vi "ultima aula labview.vi"() -> ()   [LabVIEW 2024]
uses:
  <vilib>/Instr/_visa.llb/VISA Configure Serial Port (Instr).vi
panel:
  out "output 2":dbl
  out "output 1":dbl
  out "Temperature":dbl(graph)
  out "Humicity":dbl(graph)
  in  "termination char\n(0xA = '\\n' = LF)":u8=10 format="%.0x"
  out "read buffer":string
  in  "Numeric":dbl
  in  "VISA resource name":refnum<visa-resource-name>
  in  "String":string
  in  "stop":bool
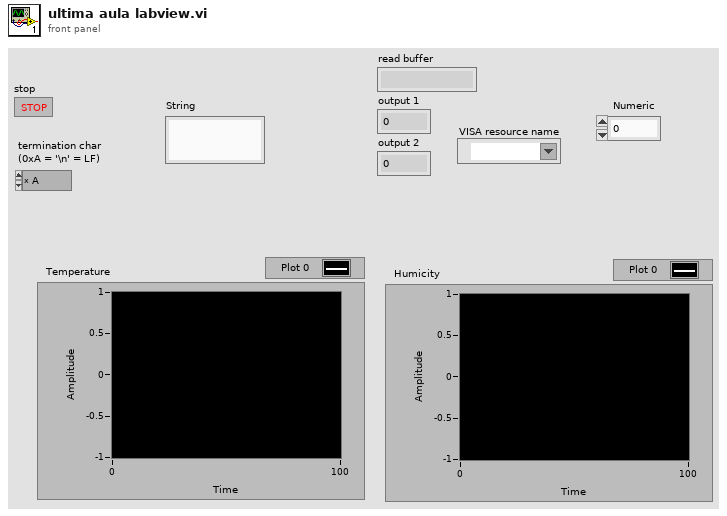
[diagram p1: front panel]
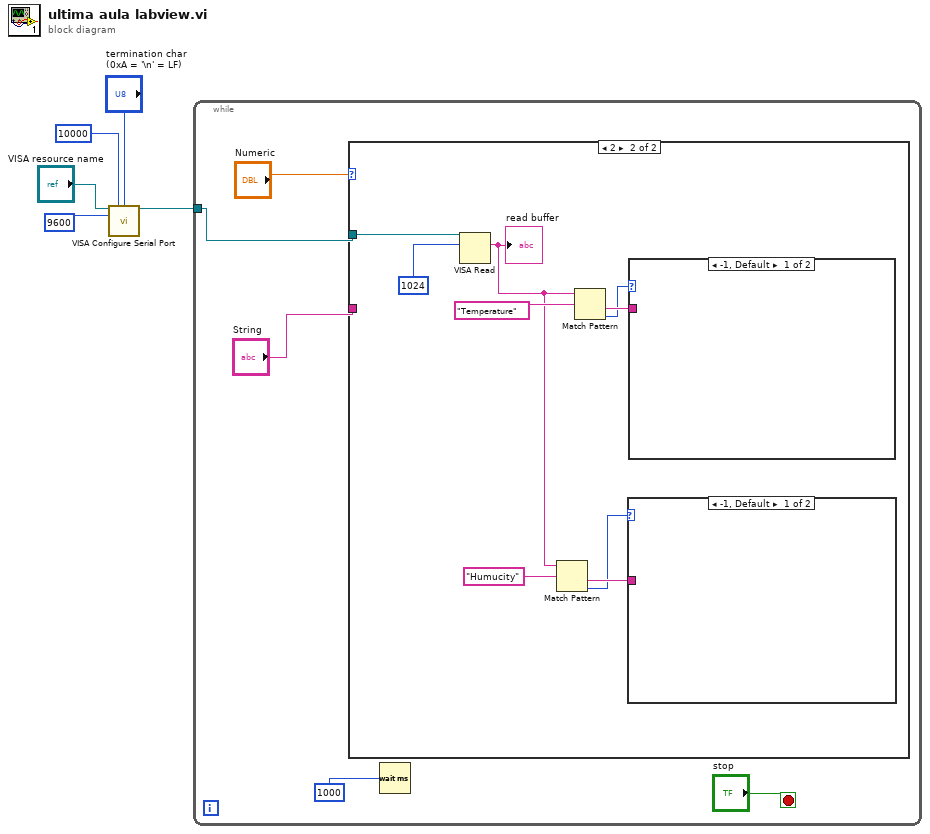
[diagram p0: block diagram]
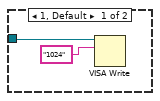
[diagram p2: hidden frame]
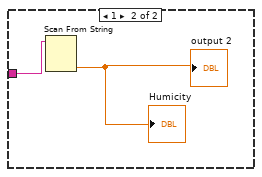
[diagram p3: hidden frame]
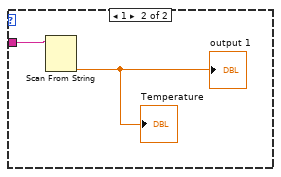
[diagram p4: hidden frame]
diagram:
  n1 = call-poly "VISA Configure Serial Port"("VISA resource name"="VISA resource name", "timeout (10sec)"=u32 10000, "termination char\n(0xA = '\\n' = LF)"="termination char\n(0xA = '\\n' = LF)", "baud rate (9600)"=u32 9600) -> ("VISA resource name out"=w4:refnum<visa-resource-name>)  [unwired: 10 in, 1 out]
  n2 = while {
    tunnel: w4 -> [w6]
    stop <- "stop" stop-if-true
    n3 = case shown="2" "Numeric" {
      tunnel: "String" -> [_ _]
      tunnel: w6 -> [w12 w21]
      frame 1, Default {
        n4 = VISA Write(VISA resource name=w12, write buffer="1024") -> ()  [unwired: 1 in, 3 out]
      }
      frame 2 {
        n5 = VISA Read(VISA resource name=w21, byte count=u32 1024) -> (read buffer=w17:string)  [unwired: 1 in, 3 out]
        "read buffer" <- w17
        n6 = Match Pattern(string=w17, regular expression="Humucity") -> (after substring=w16:string, offset past match=w13:i32)  [unwired: 1 in, 2 out]
        n7 = Match Pattern(string=w17, regular expression="Temperature") -> (after substring=w15:string, offset past match=w14:i32)  [unwired: 1 in, 2 out]
        n8 = case shown="-1, Default" w13 {
          tunnel: w16 -> [_ w22]
          frame -1, Default {
          }
          frame 1 {
            n9 = Scan From String(input string=w22) -> (output 1=→"Humicity" →"output 2":dbl)  [unwired: 4 in, 3 out]
          }
        }
        n10 = case shown="-1, Default" w14 {
          tunnel: w15 -> [_ w25]
          frame -1, Default {
          }
          frame 1 {
            n11 = Scan From String(input string=w25) -> (output 1=→"Temperature" →"output 1":dbl)  [unwired: 4 in, 3 out]
          }
        }
      }
    }
    n12 = Wait (ms)(milliseconds to wait=u32 1000) -> ()  [unwired: 1 out]
  }
